vi "Read IV.vi"() -> ()   [LabVIEW 2015]
panel:
  in  "Magnify Avg":dbl=1000.0
  out "Waveform Graph":waveform(dbl)[](graph)
  in  "Channels":string[](array[string])=["CH0", "CH1", "Avg Volts"]
  in  "Path":path=path "C:/Data/May_2016/051216/rp201905_051216.tdms"
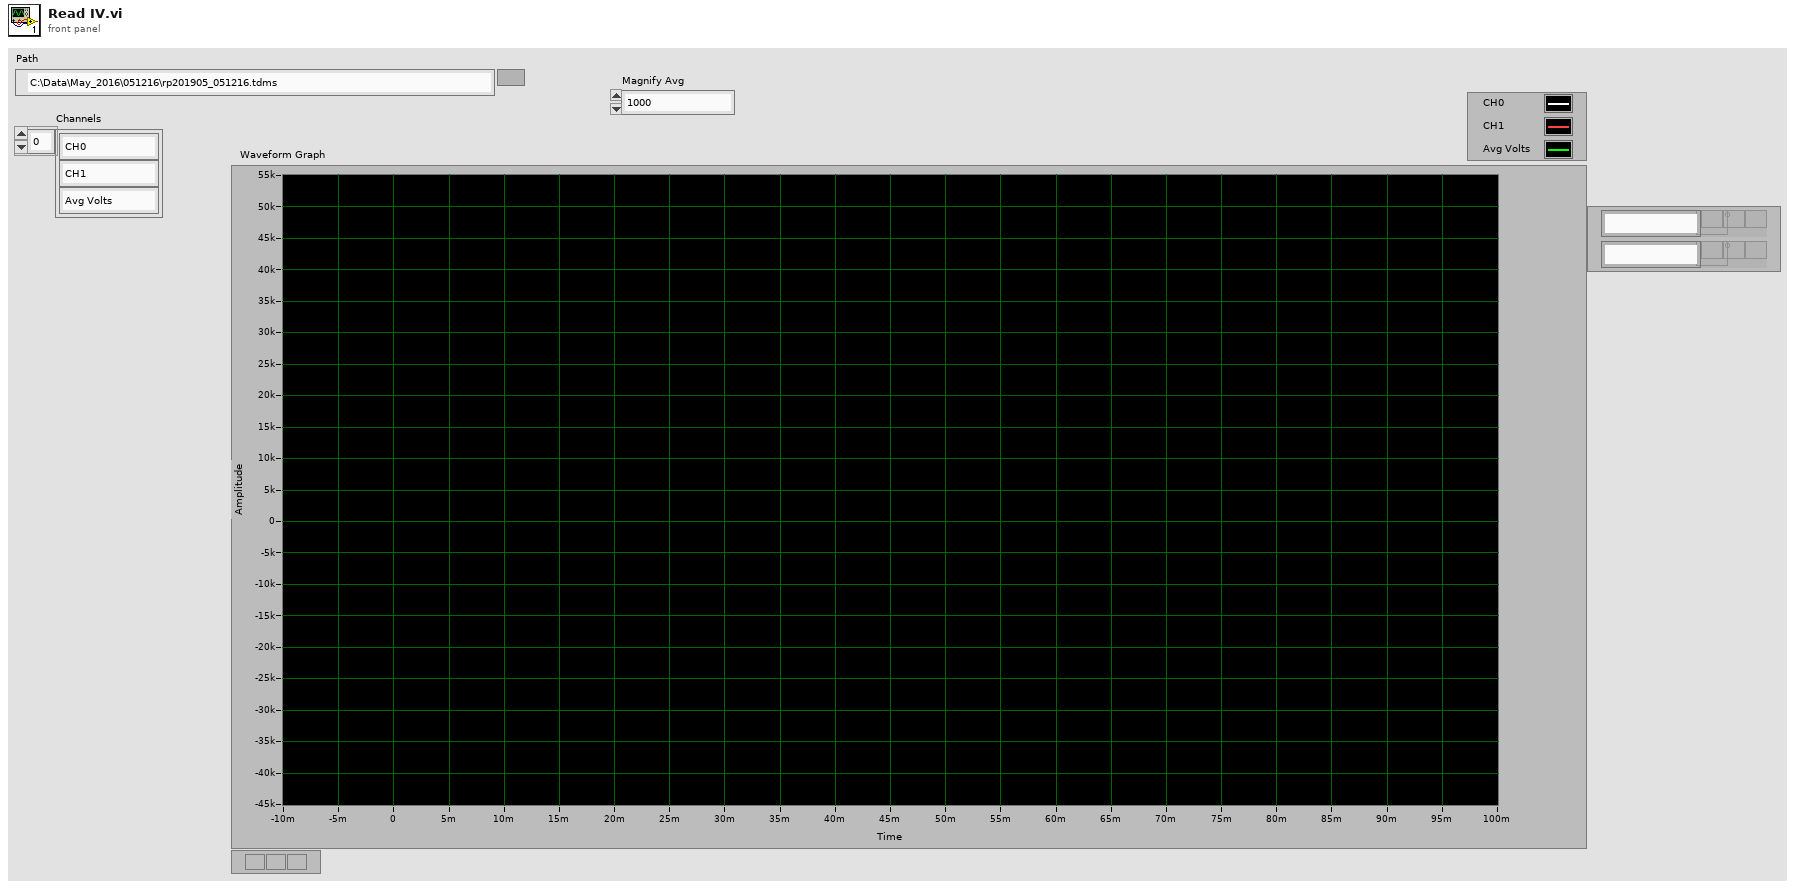
[diagram p1: front panel]
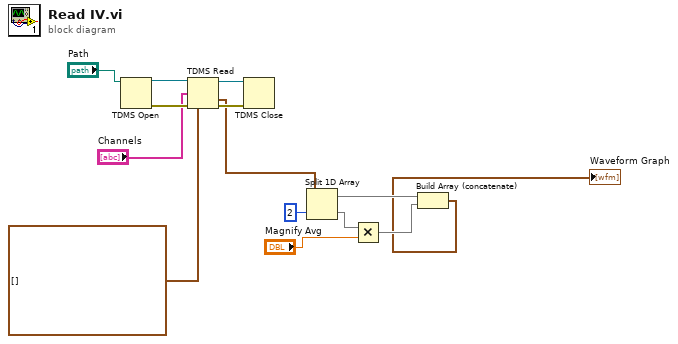
[diagram p0: block diagram]
diagram:
  n1 = TDMS Open(11:"Path") -> (0:w12:errorcluster, 3:w13:refnum<k34>)  [unwired: 6 in]
  n2 = TDMS Read(0:w13, 7:"Channels", 11:w12, 12:waveform(dbl)[] []) -> (4:w8:refnum<k34>, 10:w7:waveform(dbl)[], 15:w9:errorcluster)  [unwired: 4 in, 3 out]
  n3 = TDMS Close(8:w9, 11:w8) -> ()  [unwired: 2 out]
  n4 = Split 1D Array(array=w7, index=2) -> (first subarray=w3:waveform(dbl)[], second subarray=w5:waveform(dbl)[])
  n5 = Multiply(x=w5, y="Magnify Avg") -> (x*y=w2:waveform(dbl)[])
  n6 = Build Array (concatenate)(w3, w2) -> (→"Waveform Graph":waveform(dbl)[])
